vi "Close Command Writer.vi"(8 "error in (no error)":errorcluster, 11 "Refnum in":refnum<k21>) -> (0 "error out":errorcluster)   [LabVIEW 2016]
uses:
  HostRTCommunication/Command and Parameters.ctl
  HostRTCommunication/Commands.ctl
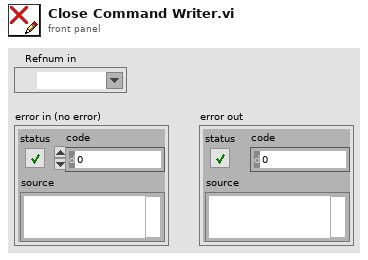
[diagram p1: front panel]
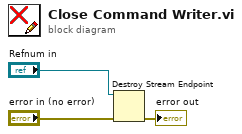
[diagram p0: block diagram]
diagram:
  n1 = Destroy Stream Endpoint(8:"error in (no error)", 11:"Refnum in") -> (0:→"error out":errorcluster)
